vi "XIPIN_Distributed_Memory_Generator_7_2.vi"   [LabVIEW 2017]
doc: "Rev 1. The LogiCORE Xilinx Distributed Memory Generator creates area and performance optimized ROM blocks, single and dual port distributed memories, and SRL16-based memories for Xilinx FPGAs. The core supersedes the previously released LogiCORE Distributed Memory core. Use this core in all new designs for supported families wherever a distributed memory is required.\n------------------------------------\n<b>Need License</b> : No"
uses:
  <vilib>/rvi/XilinxIP/XIPIN_XNode/niFpgaXIPIN.xnode
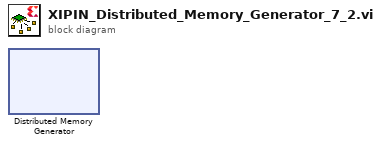
[diagram p0: block diagram]
diagram:
  n1 = xnode ("Distributed Memory Generator")() -> ()
